vi "Exemple.vi"() -> ()   [LabVIEW 2020]
uses:
  System.IO.Compression.FileSystem
panel:
  out "Current":string
  out "error out 2":errorcluster
  out "CreationTime 2":timestamp
  out "error out":errorcluster
  out "CreationTime":timestamp
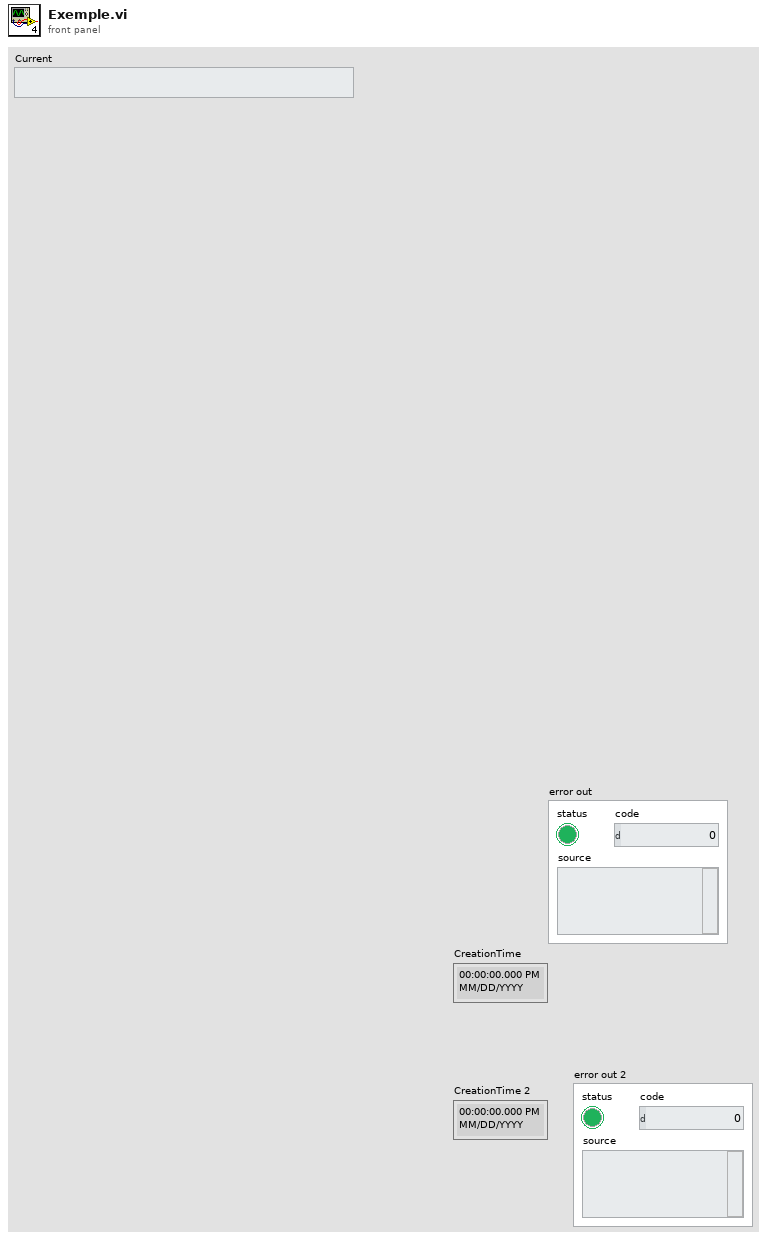
[diagram p1: front panel]
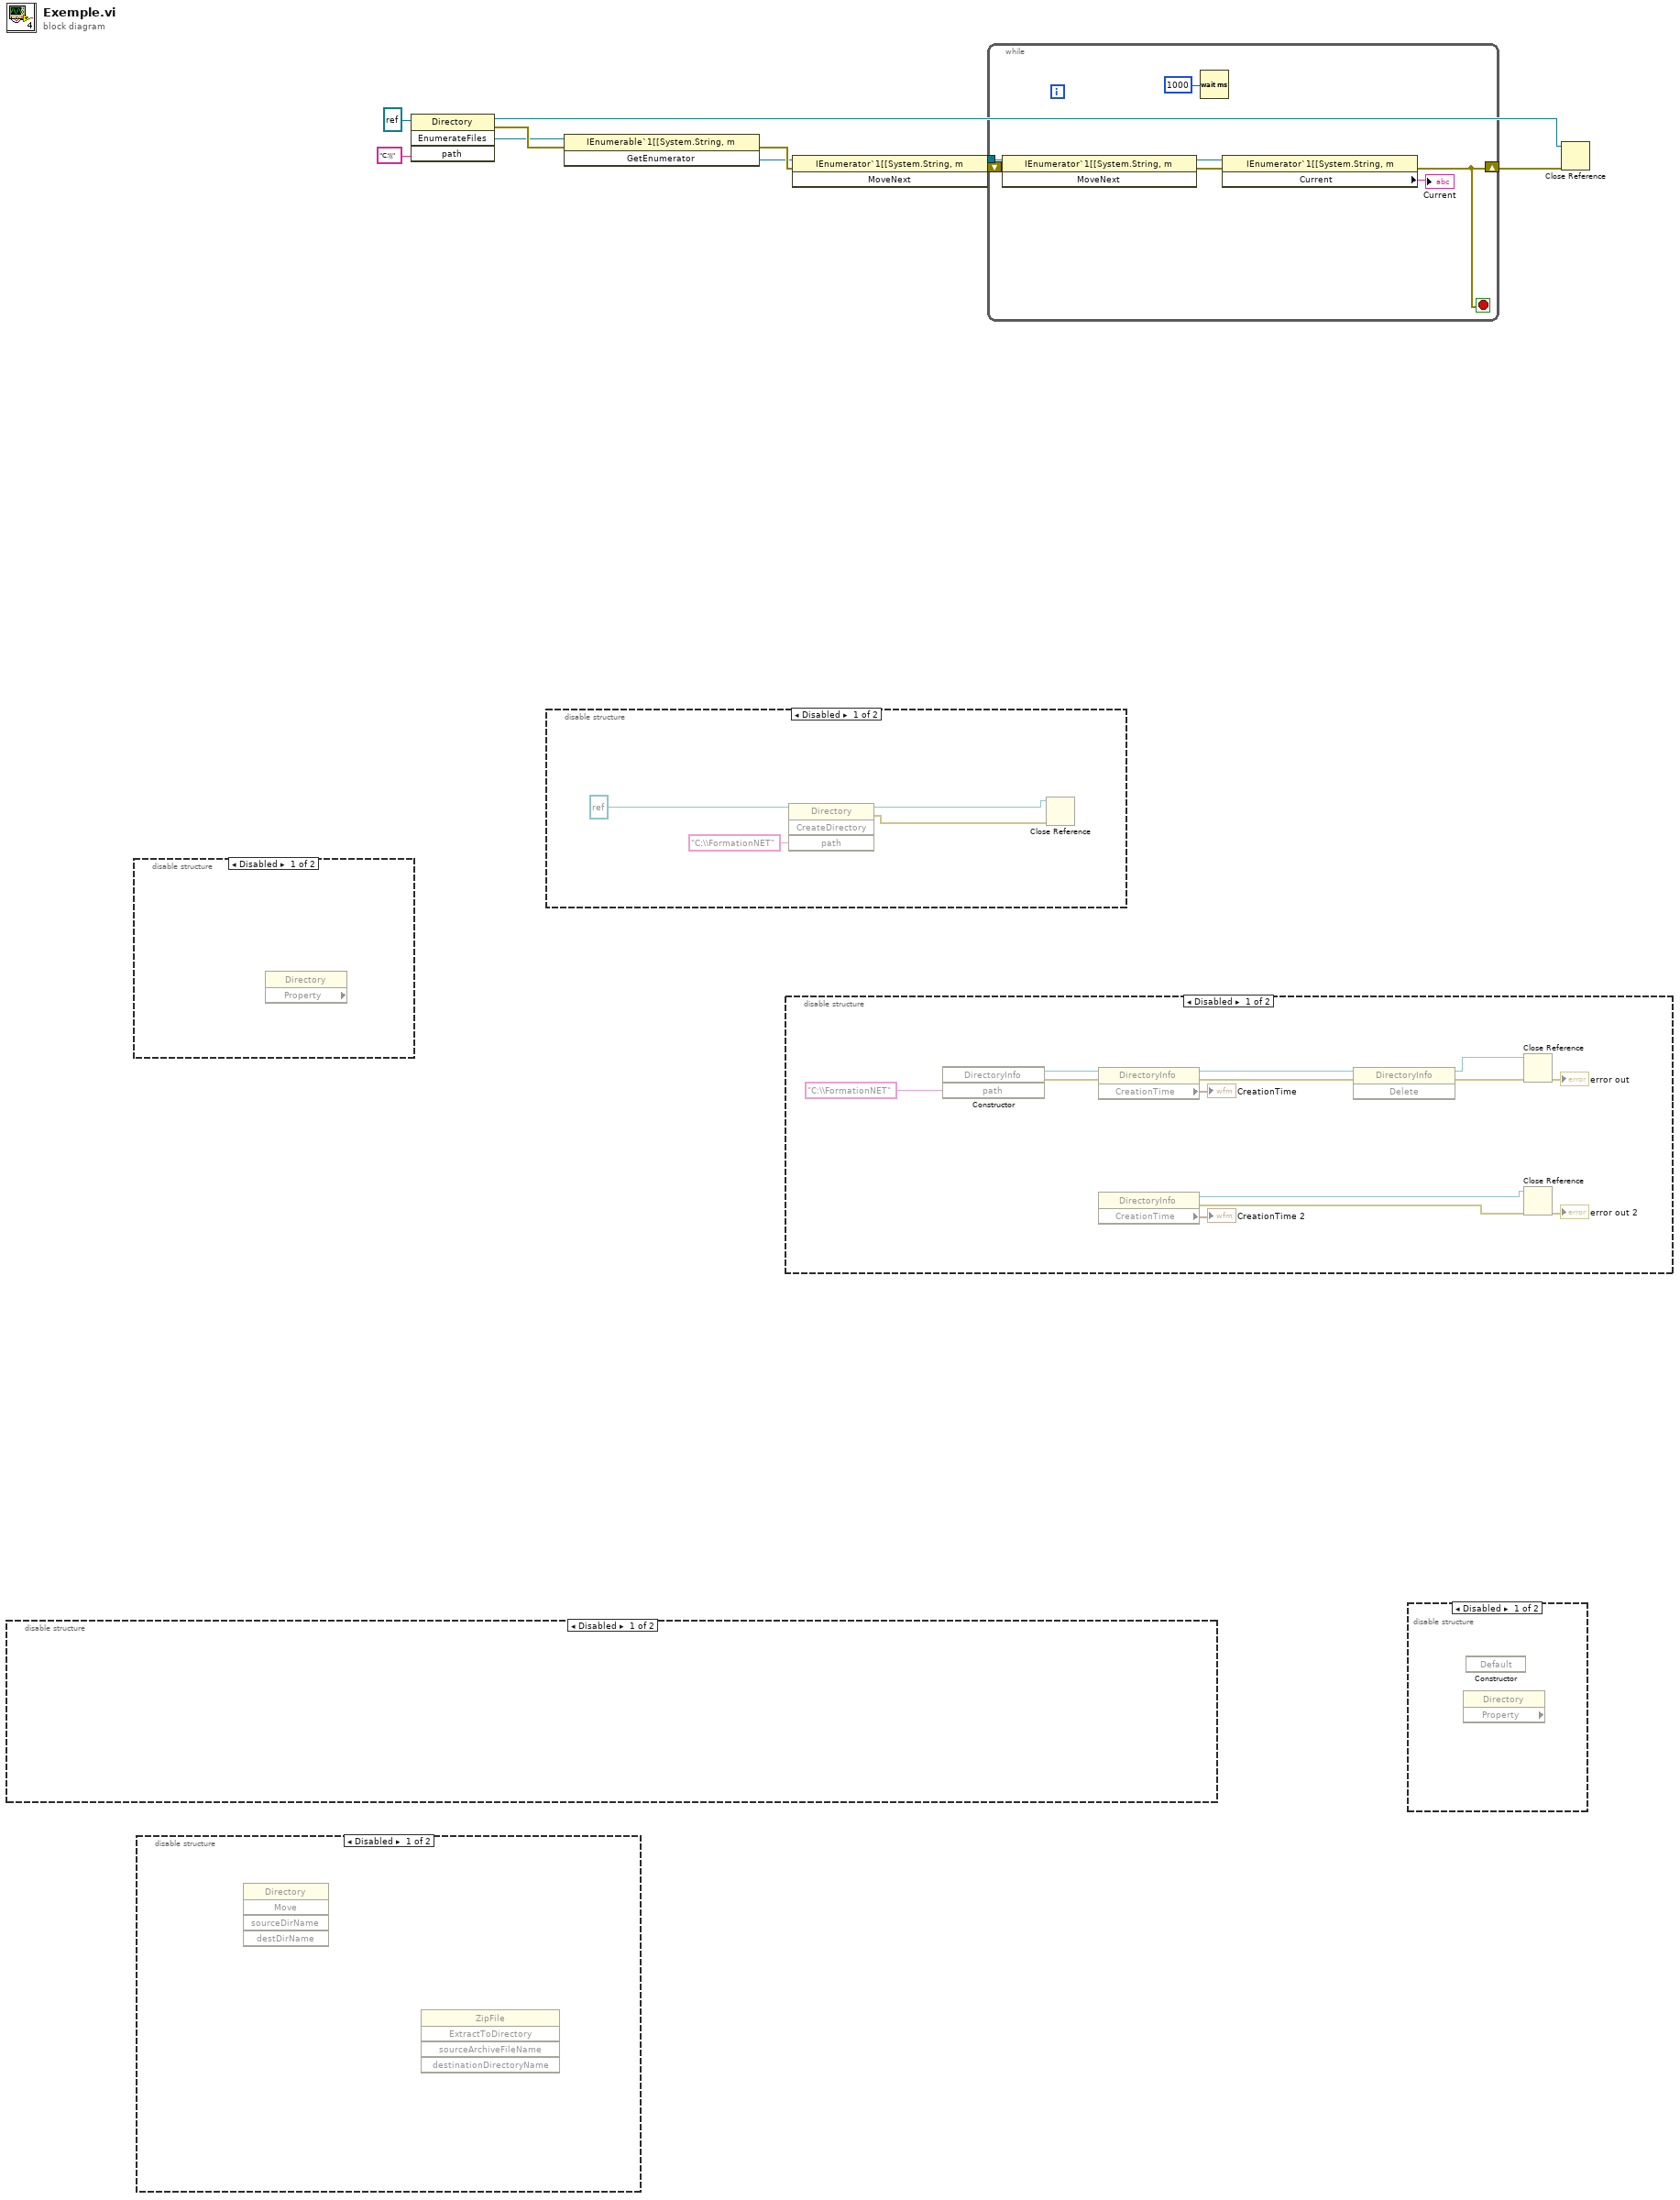
[diagram p0: block diagram]
diagram:
  n1 = disable-structure shown="Disabled" {
    frame Disabled {
    }
    frame Enabled {
    }
  }
  n2 = disable-structure shown="Disabled" {
    frame Disabled {
      n3 = property class="Directory" props=[]() -> ()  [unwired: 2 in, 3 out]
    }
    frame Enabled {
    }
  }
  n4 = disable-structure shown="Disabled" {
    frame Disabled {
      n5 = invoke class="Directory" method="Move"() -> ()  [unwired: 5 in, 5 out]
      n6 = invoke class="ZipFile" method="ExtractToDirectory"() -> ()  [unwired: 5 in, 5 out]
    }
    frame Enabled {
    }
  }
  n7 = invoke class="Directory" method="EnumerateFiles"(reference=refnum<k24> refnum, "path"="C:\\") -> (reference out=w4:refnum<k24>, error out=w8:errorcluster, "EnumerateFiles"=w7:refnum<k24>)  [unwired: 2 in, 1 out]
  n8 = disable-structure shown="Disabled" {
    frame Disabled {
      n9 = invoke class="Directory" method="CreateDirectory"(reference=refnum<k24> refnum, "path"="C:\\FormationNET") -> (reference out=w11:refnum<k24>, error out=w12:errorcluster)  [unwired: 2 in, 2 out]
      n10 = Close Reference(reference=w11, error in (no error)=w12) -> ()  [unwired: 1 out]
    }
    frame Enabled {
    }
  }
  n11 = invoke class="IEnumerable`1[[System.String, m" method="GetEnumerator"(reference=w7, error in=w8) -> (error out=w10:errorcluster, "GetEnumerator"=w9:refnum<k24>)  [unwired: 1 in, 1 out]
  n12 = disable-structure shown="Disabled" {
    frame Disabled {
      n13 = constructor class="DirectoryInfo"("path"="C:\\FormationNET") -> (reference out=w26:refnum<k24>, error out=w25:errorcluster)  [unwired: 3 in, 2 out]
      n14 = property class="DirectoryInfo"(reference=w26, error in=w25) -> (reference out=w23:refnum<k24>, error out=w22:errorcluster, "CreationTime"=→"CreationTime":timestamp)
      n15 = property class="DirectoryInfo"() -> (reference out=w16:refnum<k24>, error out=w15:errorcluster, "CreationTime"=→"CreationTime 2":timestamp)  [unwired: 2 in]
      n16 = invoke class="DirectoryInfo" method="Delete"(reference=w23, error in=w22) -> (reference out=w20:refnum<k24>, error out=w21:errorcluster)  [unwired: 1 in, 1 out]
      n17 = Close Reference(reference=w20, error in (no error)=w21) -> (error out=→"error out":errorcluster)
      n18 = Close Reference(reference=w16, error in (no error)=w15) -> (error out=→"error out 2":errorcluster)
    }
    frame Enabled {
    }
  }
  n19 = invoke class="IEnumerator`1[[System.String, m" method="MoveNext"(reference=w9, error in=w10) -> (reference out=w2:refnum<k24>, error out=w1:errorcluster)  [unwired: 1 in, 1 out]
  n20 = while {
    tunnel: w2 -> [w33]
    shift-right: [w28] -> w3
    shift-left: w1 -> [w32]
    stop <- w28 stop-if-true
    n21 = invoke class="IEnumerator`1[[System.String, m" method="MoveNext"(reference=w33, error in=w32) -> (reference out=w31:refnum<k24>, error out=w30:errorcluster)  [unwired: 1 in, 1 out]
    n22 = Wait (ms)(milliseconds to wait=u32 1000) -> ()  [unwired: 1 out]
    n23 = property class="IEnumerator`1[[System.String, m"(reference=w31, error in=w30) -> (error out=w28:errorcluster, "Current"=→"Current":string)  [unwired: 1 out]
  }
  n24 = disable-structure shown="Disabled" {
    frame Disabled {
      n25 = property class="Directory" props=[]() -> ()  [unwired: 2 in, 3 out]
      n26 = constructor class=".NET"() -> ()  [unwired: 3 in, 3 out]
    }
    frame Enabled {
    }
  }
  n27 = Close Reference(reference=w4, error in (no error)=w3) -> ()  [unwired: 1 out]
